vi "SM_AI-DAQInstrument.vi"(7 "AI TaskName":string, 8 "error in (no error)":errorcluster, 11 "DAQ Process AppData":T1) -> (0 "error out":errorcluster)   [LabVIEW 2022 SP3, in "DAQ.lvclass"]
doc: "Developed by Kevin Thompson\nkevin@thompsonengineering.net\n\nCopyright 2018-2020\nThompson Engineering, LLC"
uses:
  DAQ.lvclass
  Process_DAQ SM AppData--cluster.ctl
  DataTypes/TD DAQ Settings--cluster.ctl
  DataTypes/TD DI Instrument Settings--cluster.ctl
  DataTypes/TD AI Instrument Settings--cluster.ctl
  DataTypes/TD AI InstSettings--cluster.ctl
  TD SimAI Ranges--cluster.ctl
  <vilib>/TELLC/Dynamic CVT API/TD Dynamic CVT DVR--ref.ctl
  Support/DataQueues/DataTypes/DataQ SelectType--enum.ctl
  DAQ.lvclass/DAQ.ctl
  TD local raw AI Data--cluster.ctl
  DataTypes/AsyncMsg_DAQ--enum.ctl
  DataTypes/TD DaqState--enum.ctl
  <vilib>/DAQmx/read.llb/DAQmx Read (Analog 2D DBL NChan NSamp).vi
  Accessors/Get Dependency.vi
  Util/CONST AI TaskIO KeyName.vi
  <vilib>/TELLC/Dynamic CVT API/Get Dynamic CVT Data.vi
  <vilib>/DAQmx/miscellaneous.llb/DAQmx Fill In Error Info.vi
  Support/DataQueues/DataQueues.lvclass
  DAQ_Common/Lib/ErrorHandler/ErrorHandler.lvclass
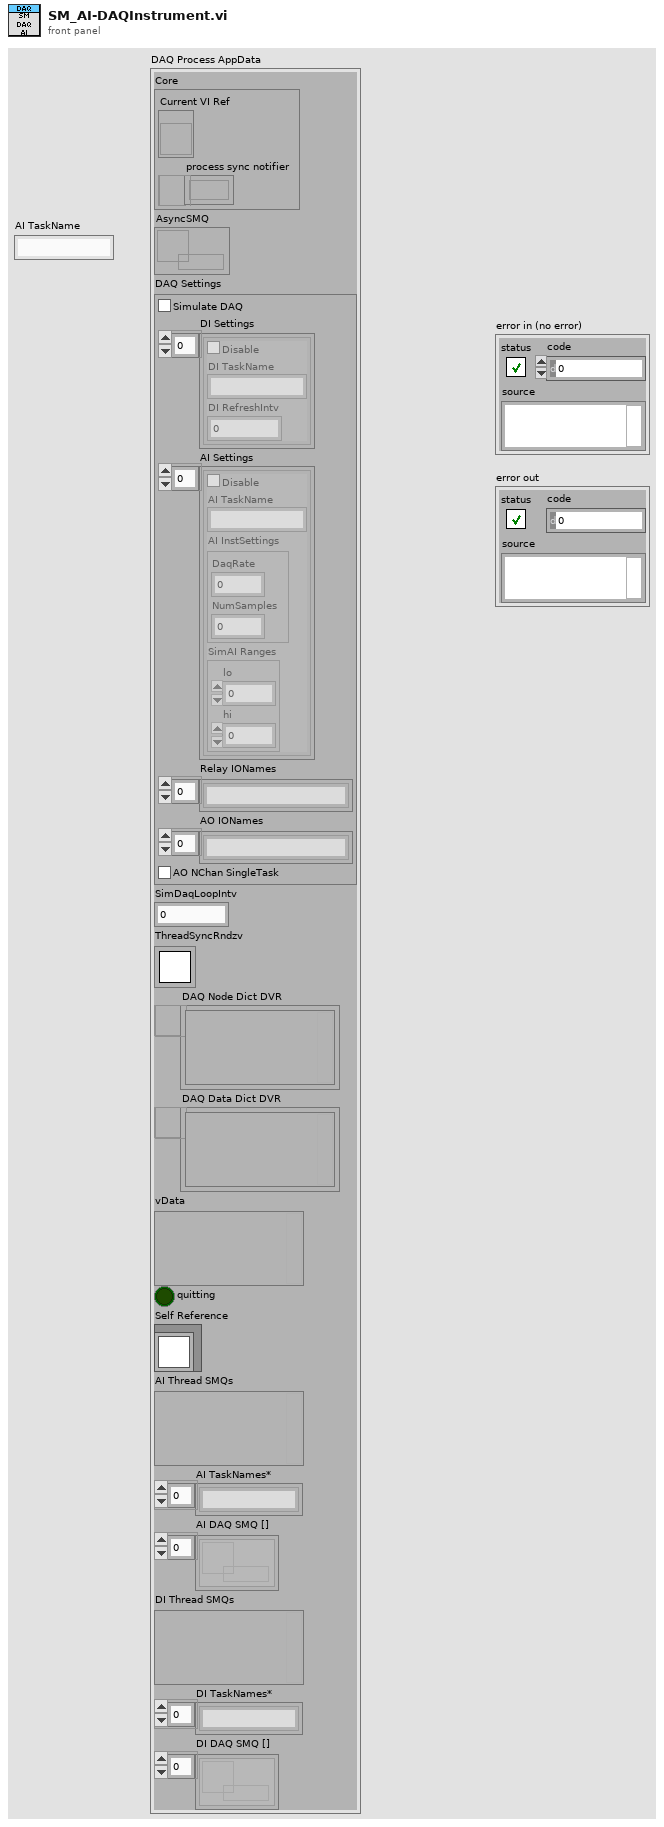
[diagram p1: front panel]
types:
  T1 = typedef "DAQ.lvclass/Process_DAQ SM AppData--cluster.ctl" = cluster{"Core":cluster{"Current VI Ref":refnum<vi>, "process sync notifier":refnum<notifier>}, "AsyncSMQ":refnum<queue>, "DAQ Settings":T2, "SimDaqLoopIntv":i32, "ThreadSyncRndzv":T7, "DAQ Node Dict DVR":T8, "DAQ Data Dict DVR":T8, "vData":variant, "quitting":bool, "Self Reference":refnum<class "DAQ.lvclass">, "AI Thread SMQs":variant, "AI TaskNames*":string[], "AI DAQ SMQ []":refnum<queue>[], "DI Thread SMQs":variant, "DI TaskNames*":string[], "DI DAQ SMQ []":refnum<queue>[]}
  T2 = typedef "DAQ.lvclass/TD DAQ Settings--cluster.ctl" = cluster{"Simulate DAQ":bool, "DI Settings":T3[], "AI Settings":T4[], "Relay IONames":string[], "AO IONames":string[], "AO NChan SingleTask":bool}
  T3 = typedef "DAQ.lvclass/TD DI Instrument Settings--cluster.ctl" = cluster{"Disable":bool, "DI TaskName":string, "DI RefreshIntv":i32}
  T4 = typedef "DAQ.lvclass/TD AI Instrument Settings--cluster.ctl" = cluster{"Disable":bool, "AI TaskName":string, "AI InstSettings":T5, "SimAI Ranges":T6}
  T5 = typedef "DAQ.lvclass/TD AI InstSettings--cluster.ctl" = cluster{"DaqRate":dbl, "NumSamples":i32}
  T6 = typedef "DAQ.lvclass/TD SimAI Ranges--cluster.ctl" = cluster{"lo":dbl, "hi":dbl}
  T7 = typedef "Rendezvous RefNum" = refnum<k1>
  T8 = typedef "TD Dynamic CVT DVR--ref.ctl" = refnum<data-value>
  T9 = enum32{"Invalid", "Standard", "Closed", "Hidden", "Minimized", "Maximized"}
  T10 = cluster{"UpdateUIControl Ev":refnum<user-event>, "stop process Ev":refnum<user-event>, "change mode Ev":refnum<user-event>}
  T11 = typedef "DataQueues.lvclass/DataQ SelectType--enum.ctl" = enum16{"MainProcess", "LogEngine", "LocalDAQThread"}
  T12 = typedef "DAQ.lvclass/TD local raw AI Data--cluster.ctl" = cluster{"TimeStamp_(s)":dbl, "data":dbl[][]}
  T13 = typedef "DAQ.lvclass/AsyncMsg_DAQ--enum.ctl" = enum16{"DAQ.SendAI_InstSettings"}
  T14 = typedef "DAQ.lvclass/TD DaqState--enum.ctl" = enum16{"Unknown", "Stopped", "Running", "Error"}
  T15 = typedef "DAQ.lvclass/TD AI local thread params--clustser.ctl" = cluster{"AI IONames":string[], "DAQ running":bool, "RawAIDataQ":T16, "AI Local CmdQ":refnum<queue>, "AI TaskName":string, "AI SMQ":refnum<queue>, "AI Settings":T4, "MainProc_ScanDataQ":T17, "Logger_ScanDataQ":T17, "DAQ Task Start Time":timestamp}
  T16 = typedef "DataQueues.lvclass/Analog DataSet MultiRow--QRef.ctl" = refnum<queue>
  T17 = typedef "DataQueues.lvclass/Analog DataSet MultiRow & ChanNames--QRef.ctl" = refnum<queue>
  T18 = cluster{"DAQ Process AppData":T1, "AI thread params":T15}
  T19 = typedef "Type Descriptor Enumeration__ogtk.ctl" = enum8{"<Null>", "I8", "I16", "I32", "I64", "U8", "U16", "U32", "U64", "SGL", "DBL", "EXT", "CSG", "CDB", "CXT", "0x0F", "0x10", "0x11", "0x12", "0x13", "0x14", "Enum U8", "Enum U16", "Enum U32", "Enum U64", "SGL PQ", "DBL PQ", "EXT PQ", "CSG PQ", "CDB PQ", "CXT PQ", "0x1F", "0x20", "Boolean", "0x22", "0x23", "0x24", "0x25", "0x26", "0x27", "0x28", "0x29", "0x2A", "0x2B", "0x2C", "0x2D", "0x2E", "0x2F", "String", "0x31", "Path", "Pict", "0x34", "0x35", "0x36", "DAQ", "0x38", "0x39", "0x3A", "0x3B", "0x3C", "0x3D", "0x3E", "0x3F", "Array", "0x41", "0x42", "0x43", "0x44", "0x45", "0x46", "0x47", "0x48", "0x49", "0x4A", "0x4B", "0x4C", "0x4D", "0x4E", "0x4F", "Cluster", "0x51", "0x52", "Variant", "Waveform", "0x55", "0x56", "0x57", "0x58", "0x59", "0x5A", "0x5B", "0x5C", "0x5D", "0x5E", "Fixed Point", "0x60", "0x61", "0x62", "0x63", "0x64", "0x65", "0x66", "0x67", "0x68", "0x69", "0x6A", "0x6B", "0x6C", "0x6D", "0x6E", "0x6F", "Refnum", "0x71", "0x72", "Set Collection", "Map Collection"}
  T20 = typedef "DAQ.lvclass/TD DAQ Device--enum.ctl" = enum16{"DI", "DO", "AIVolt", "AICurr", "AILoRes", "AO"}
  T21 = typedef "DAQ.lvclass/Dependency--cluster.ctl" = cluster{"DataQueues":refnum<class "DataQueues.lvclass">}
  T22 = cluster{"AI InstSettings":T5, "AI TaskName":string}
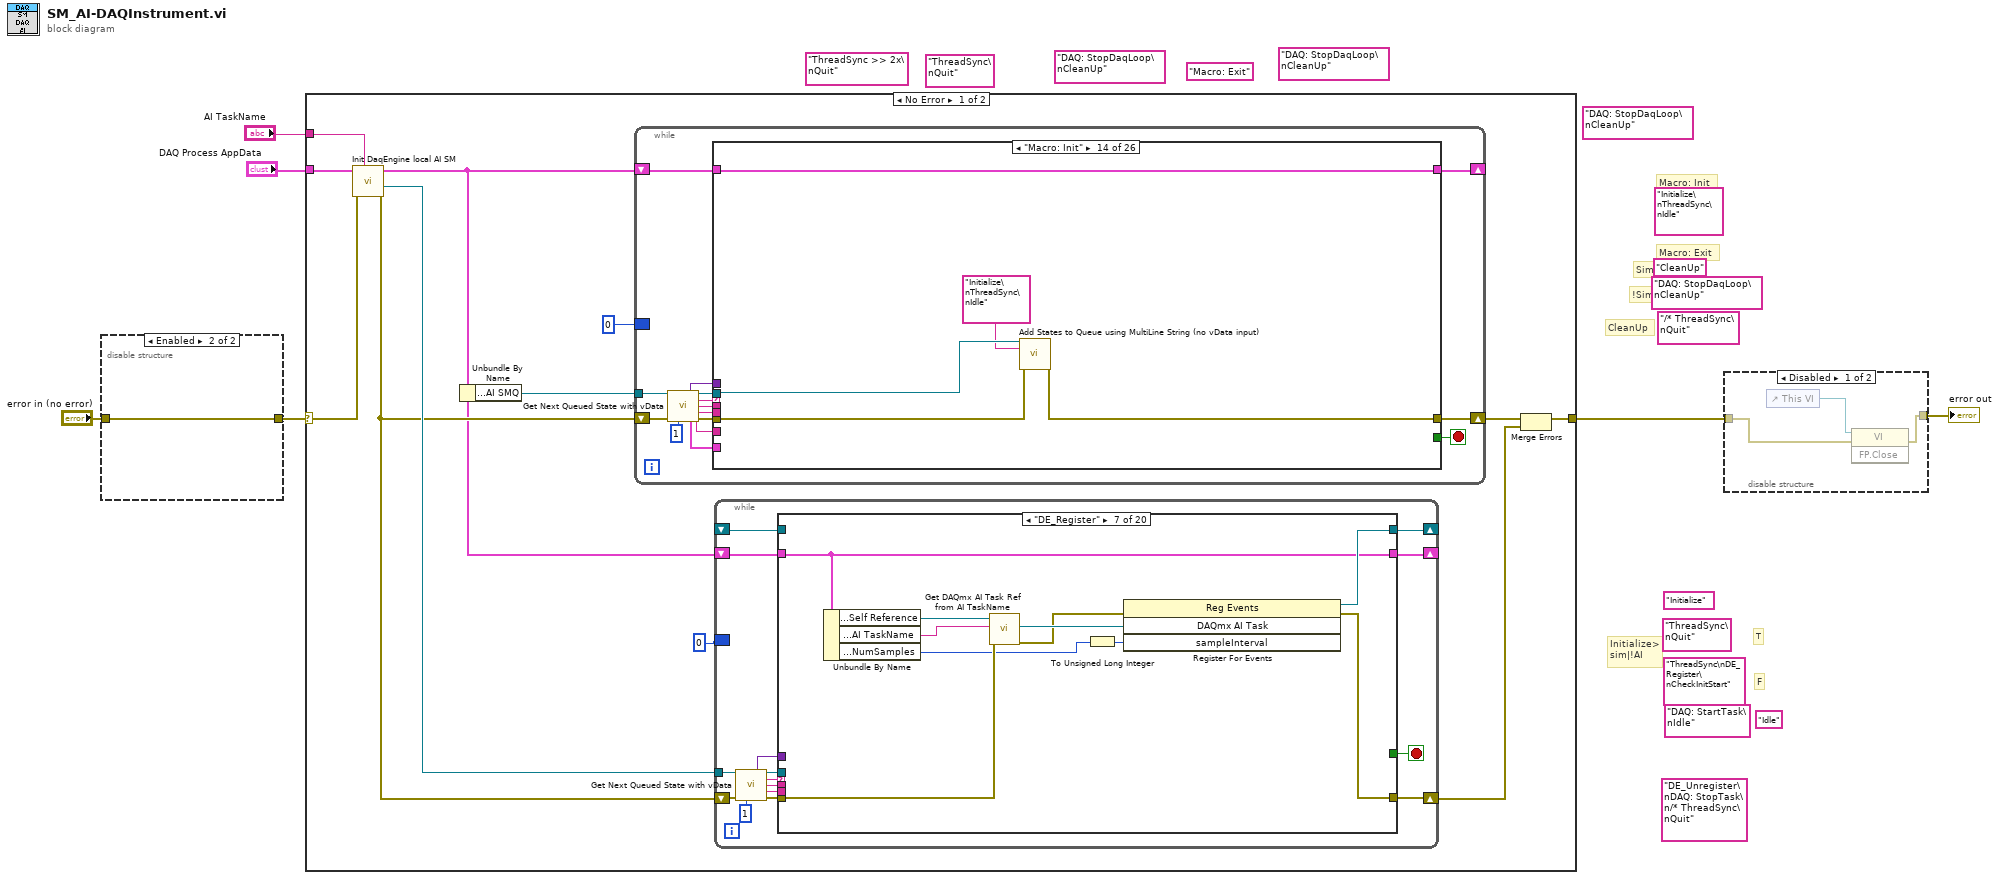
[diagram p0: block diagram]
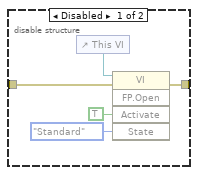
[diagram p3: hidden frame]
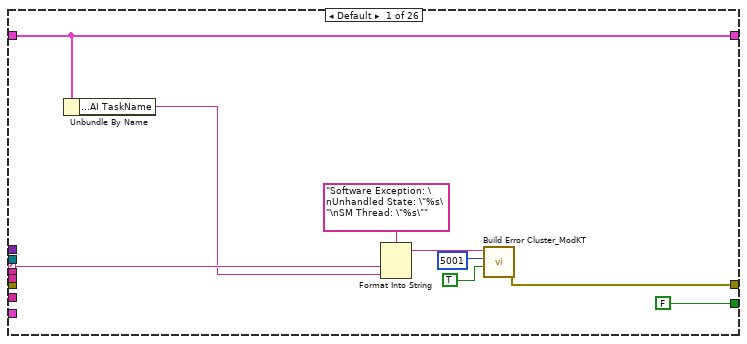
[diagram p4: hidden frame]
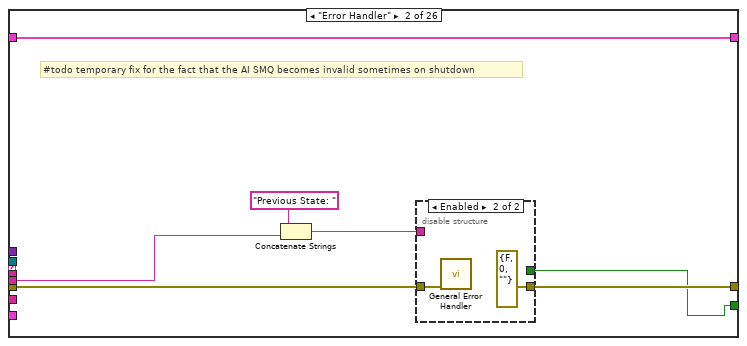
[diagram p5: hidden frame]
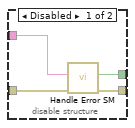
[diagram p6: hidden frame]
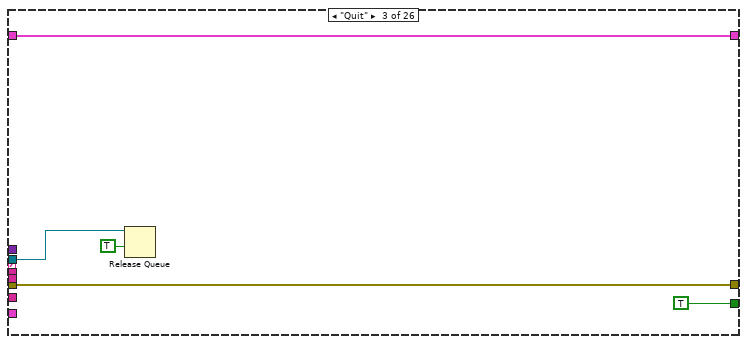
[diagram p7: hidden frame]
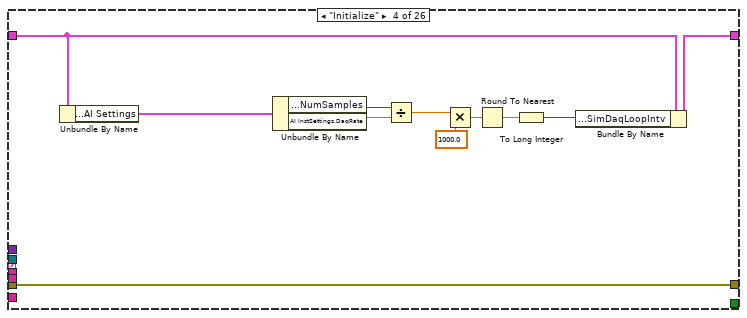
[diagram p8: hidden frame]
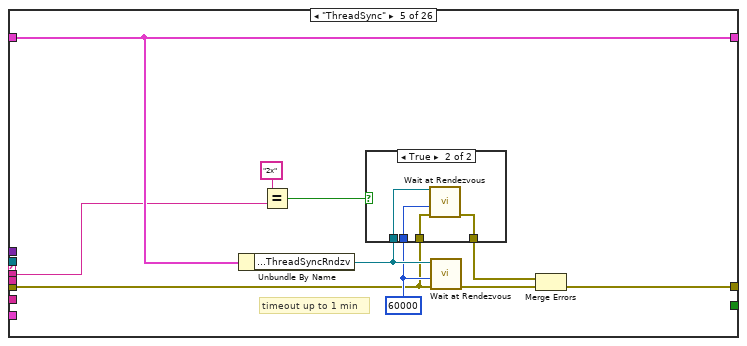
[diagram p9: hidden frame]
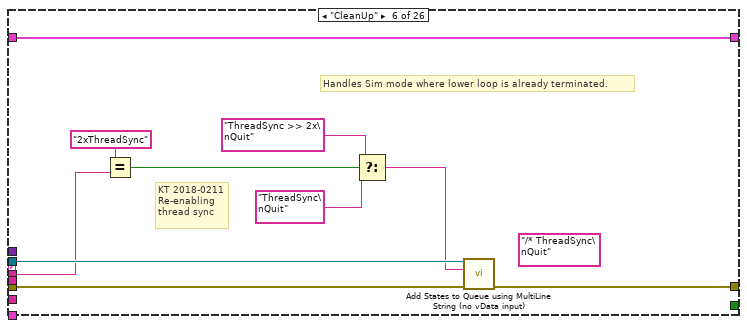
[diagram p11: hidden frame]
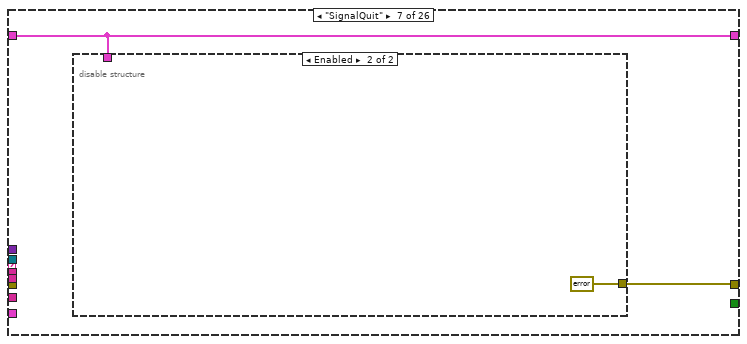
[diagram p12: hidden frame]
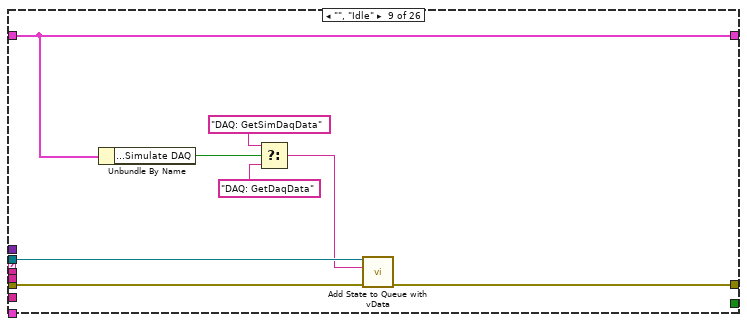
[diagram p15: hidden frame]
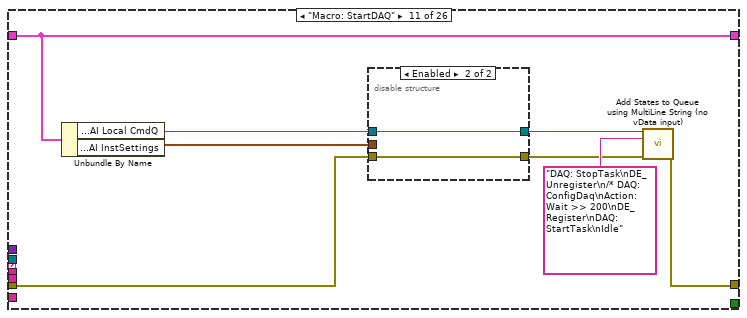
[diagram p17: hidden frame]
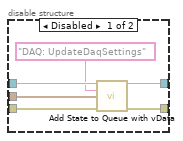
[diagram p18: hidden frame]
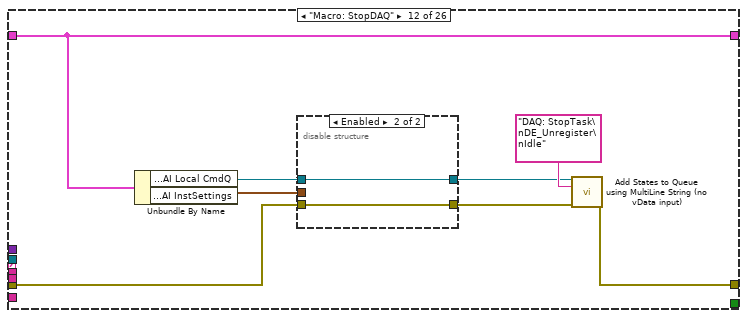
[diagram p19: hidden frame]
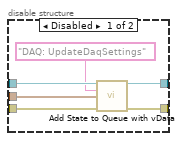
[diagram p20: hidden frame]
diagram:
  (unwired) "ThreadSync >> 2x\nQuit" ("states in")
  (unwired) "ThreadSync\nQuit" ("states in")
  (unwired) "DAQ: StopDaqLoop\nCleanUp"
  (unwired) "Macro: Exit"
  (unwired) "DAQ: StopDaqLoop\nCleanUp"
  (unwired) "DAQ: StopDaqLoop\nCleanUp"
  (unwired) "Idle"
  (unwired) "DAQ: StartTask\nIdle"
  (unwired) "ThreadSync\nDE_Register\nCheckInitStart"
  (unwired) "DE_Unregister\nDAQ: StopTask\n/* ThreadSync\nQuit" ("states in")
  (unwired) "Initialize" ("states in")
  (unwired) "ThreadSync\nQuit"
  (unwired) "/* ThreadSync\nQuit" ("states in")
  (unwired) "DAQ: StopDaqLoop\nCleanUp"
  (unwired) "CleanUp"
  (unwired) "Initialize\nThreadSync\nIdle"
  # "F"
  # "T"
  # "Initialize>\nsim|!AI"
  # "CleanUp"
  # "!Sim"
  # "Sim"
  # "Macro: Init"
  # "Macro: Exit"
  n1 = disable-structure shown="Enabled" {
    disable-tunnel: "error in (no error)" -> [w8 w12]
    disable-tunnel: [w7 w12] -> w1
    frame Disabled {
      n2 = control-ref of="This VI"() -> (w11:refnum<vi>)
      n3 = invoke class="VI" method="FP.Open"(reference=w11, error in=w8, "Activate"=TRUE ("Activate?"), "State"=T9."Standard") -> (error out=w7:errorcluster)  [unwired: 1 in, 4 out]
    }
    frame Enabled {
    }
  }
  n4 = case shown="No Error" w1 {
    selector: w1 -> [w22 w615]
    tunnel: [w20 w615] -> w4
    tunnel: "DAQ Process AppData" -> [w16 _]
    tunnel: "AI TaskName" -> [w15 _]
    frame No Error {
      n5 = call "Init DaqEngine local AI SM.vi"("AI TaskName"=w15, "error in (no error)"=w22, "DAQ Process AppData"=w16) -> ("error out"=w21:errorcluster, "local LoopCmdQ"=w23:refnum<queue>, "DaqProces AI AppData+"=w17:T18)  [unwired: 6 in]
      n6 = Unbundle By Name(w17) -> ("AI thread params.AI SMQ"=w14:refnum<queue>)
      n7 = while {
        shift-right: [w29] -> _
        shift-left: w17 -> [w38]
        shift-right: [w32] -> w24
        shift-left: w21 -> [w31]
        tunnel: w14 -> [w28]
        border: u32 0 -> [_]
        stop <- w34 stop-if-true
        n8 = call <vilib>:"Get Next Queued State with vData.vi"("queue in"=w28, "error in (no error)"=w31, "timeout (100)"=1) -> ("vData out"=w35:variant, "queue out"=w30:refnum<queue>, "Next State"=w37:string, "queued msg"=w36:string, "Prev State"=w25:string, "RemainingElements"=w27:cluster{"state":string, "vData":variant}[], "error out"=w33:errorcluster)  [unwired: 6 in]
        n9 = case shown="\"Macro: Init\"" w37 {
          selector: w37 -> [w42 _ _ _ _ _ _ _ _ _ _ _ _ _ _ _ _ _ _ _ _ _ _ _ _ _]
          tunnel: w38 -> [w40 w54 w65 w75 w86 w101 w102 w106 w113 w117 w118 w134 w155 w186 w193 w202 w228 w231 w235 w248 w260 w316 w320 w327 w328 w333]
          tunnel: w36 -> [_ _ _ _ w78 w97 _ _ _ _ _ _ _ _ _ _ _ _ _ _ _ _ _ w326 _ _]
          tunnel: w35 -> [_ _ _ _ _ _ _ _ _ _ _ _ w151 _ _ w203 _ _ _ _ _ _ _ _ w331 w336]
          tunnel: w25 -> [_ _ _ _ _ _ _ _ _ _ _ _ _ _ _ _ _ _ _ _ _ _ _ _ _ _]
          tunnel: [FALSE w48 TRUE _ _ _ _ _ _ _ _ _ _ _ _ _ _ _ _ _ _ _ _ _ _ _] -> w34
          tunnel: w33 -> [_ w51 w64 w67 w82 w99 _ w107 w112 w116 w120 w135 w152 w189 w194 w199 w227 w232 w245 w247 w273 w317 w319 w321 w330 w337]
          tunnel: [w41 w49 w64 w67 w81 w100 w103 w107 w114 w116 w119 w136 w153 w187 w195 w200 w227 w233 w245 w246 w272 w315 w319 w322 w329 w335] -> w32
          tunnel: w30 -> [_ _ w61 _ _ w98 _ _ w115 _ _ _ _ w188 w196 w204 _ _ _ _ _ _ _ _ _ _]
          tunnel: [w40 w54 w65 w76 w86 w101 w102 w106 w113 w117 w118 w134 w154 w186 w193 w201 w228 w231 w244 w248 w260 w316 w320 w327 w328 w334] -> w29
          tunnel: w27 -> [_ _ _ _ _ _ _ _ _ _ _ _ _ _ _ _ _ _ _ _ _ _ _ _ _ _]
          tunnel: w25 -> [_ w50 _ _ _ _ _ _ _ _ _ _ _ _ _ _ _ _ _ _ _ _ _ _ _ _]
          frame Default {
            n10 = Unbundle By Name(w40) -> ("AI thread params.AI TaskName"=w39:string)
            n11 = Format Into String(format string="Software Exception: \nUnhandled State: \"%s\"\nSM Thread: \"%s\"", w42, w39) -> (resulting string=w43:string)  [unwired: 2 in, 1 out]
            n12 = call <vilib>:"Build Error Cluster_ModKT .vi"("Prepend String (\"\")"=w43, "code"=5001, "error? (F)"=TRUE ("error?")) -> ("error out"=w41:errorcluster)  [unwired: 4 in, 1 out]
          }
          frame "Error Handler" {
            # "#todo temporary fix for the fact that the AI SMQ becomes invalid sometimes on shutdown"
            n13 = Concatenate Strings("Previous State: ", w50) -> (w53:string)
            n14 = disable-structure shown="Enabled" {
              disable-tunnel: w53 -> [w58 _]
              disable-tunnel: w51 -> [w57 w60]
              disable-tunnel: [w56 errorcluster {"status"=FALSE, "code"=0, "source"=""} ("error constant")] -> w49
              disable-tunnel: [w55 _] -> w48
              frame Disabled {
                n15 = call "Handle Error SM.vi"("error in (no error)"=w57, "CustomMessage"=w58) -> ("error out"=w56:errorcluster, "Shutdown?"=w55:bool)  [unwired: 7 in, 1 out]
              }
              frame Enabled {
                n16 = call <vilib>:"General Error Handler.vi"("error in (no error)"=w60) -> ()  [unwired: 10 in, 5 out]
              }
            }
          }
          frame "Quit" {
            n17 = Release Queue(queue=w61, force destroy? (F)=TRUE) -> ()  [unwired: 1 in, 3 out]
          }
          frame "Initialize" {
            n18 = Unbundle By Name(w75) -> ("AI thread params.AI Settings"=w66:T4)
            n19 = Unbundle By Name(w66) -> ("AI InstSettings.NumSamples"=w69:i32, "AI InstSettings.DaqRate"=w68:dbl)
            n20 = Divide(x=w69, y=w68) -> (x/y=w71:dbl)
            n21 = Multiply(x=w71, y=1000.0) -> (x*y=w74:dbl)
            n22 = Round To Nearest(number=w74) -> (nearest integer value=w72:dbl)
            n23 = To Long Integer(number=w72) -> (32bit integer=w70:i32)
            n24 = Bundle By Name(cluster=w75, "DAQ Process AppData.SimDaqLoopIntv"=w70) -> (w76:T18)
          }
          frame "ThreadSync" {
            w83 = 60000 ("ms timeout (-1)")
            # "timeout up to 1 min"
            n25 = Unbundle By Name(w86) -> ("DAQ Process AppData.ThreadSyncRndzv"=w84:T7)
            n26 = Equal?(x="2x", y=w78) -> (x = y?=w77:bool)
            n27 = case shown="True" w77 {
              tunnel: w84 -> [_ w91]
              tunnel: w83 -> [_ w90]
              tunnel: w82 -> [w87 w89]
              tunnel: [w87 w88] -> w80
              frame False {
              }
              frame True {
                n28 = call <vilib>:"Wait at Rendezvous.vi"("error in (no error)"=w89, "ms timeout (-1)"=w90, "rendezvous"=w91) -> ("error out"=w88:errorcluster)  [unwired: 2 in, 2 out]
              }
            }
            n29 = call <vilib>:"Wait at Rendezvous.vi"("error in (no error)"=w82, "ms timeout (-1)"=w83, "rendezvous"=w84) -> ("error out"=w85:errorcluster)  [unwired: 2 in, 2 out]
            n30 = Merge Errors(w80, w85) -> (w81:errorcluster)
          }
          frame "CleanUp" {
            (unwired) "/* ThreadSync\nQuit" ("states in")
            # "Handles Sim mode where lower loop is already terminated."
            # "KT 2018-0211\nRe-enabling\nthread sync"
            n31 = Equal?(x="2xThreadSync", y=w97) -> (x = y?=w95:bool)
            n32 = Select(t="ThreadSync >> 2x\nQuit" ("states in"), s=w95, f="ThreadSync\nQuit" ("states in")) -> (s? t:f=w92:string)
            n33 = call <vilib>:"Add States to Queue using MultiLine String (no vData input).vi"("queue in"=w98, "states in"=w92, "error in"=w99) -> ("error out"=w100:errorcluster)  [unwired: 10 in, 2 out]
          }
          frame "SignalQuit" {
            n34 = disable-structure shown="Enabled" {
              disable-tunnel: [w104 errorcluster {"status"=FALSE, "code"=0, "source"=""} ("error constant")] -> w103
              disable-tunnel: w102 -> [_ _]
              frame Disabled {
              }
              frame Enabled {
              }
            }
          }
          frame "CheckTimer" {
            # "NoOp"
          }
          frame "", "Idle" {
            n35 = Unbundle By Name(w113) -> ("DAQ Process AppData.DAQ Settings.Simulate DAQ"=w111:bool)
            n36 = Select(t="DAQ: GetSimDaqData" ("state"), s=w111, f="DAQ: GetDaqData" ("state")) -> (s? t:f=w108:string)
            n37 = call <vilib>:"Add State to Queue with vData.vi"("queue in"=w115, "state in"=w108, "error in"=w112) -> ("error out"=w114:errorcluster)  [unwired: 9 in, 3 out]
          }
          frame "------ Macro ------" {
          }
          frame "Macro: StartDAQ" {
            n38 = Unbundle By Name(w118) -> ("AI thread params.AI Local CmdQ"=w124:refnum<queue>, "AI thread params.AI Settings.AI InstSettings"=w125:T5)
            n39 = disable-structure shown="Enabled" {
              disable-tunnel: w124 -> [w131 w133]
              disable-tunnel: w125 -> [w129 _]
              disable-tunnel: [w128 w133] -> w121
              disable-tunnel: [w127 w132] -> w122
              disable-tunnel: w120 -> [w126 w132]
              frame Disabled {
                n40 = call <vilib>:"Add State to Queue with vData.vi"("queue in"=w131, "state in"="DAQ: UpdateDaqSettings", "vData (\"\")"=w129, "error in"=w126) -> ("queue out"=w128:refnum<queue>, "error out"=w127:errorcluster)  [unwired: 8 in, 2 out]
              }
              frame Enabled {
              }
            }
            n41 = call <vilib>:"Add States to Queue using MultiLine String (no vData input).vi"("queue in"=w121, "states in"="DAQ: StopTask\nDE_Unregister\n/* DAQ: ConfigDaq\nAction: Wait >> 200\nDE_Register\nDAQ: StartTask\nIdle", "error in"=w122) -> ("error out"=w119:errorcluster)  [unwired: 10 in, 2 out]
          }
          frame "Macro: StopDAQ" {
            n42 = Unbundle By Name(w134) -> ("AI thread params.AI Local CmdQ"=w141:refnum<queue>, "AI thread params.AI Settings.AI InstSettings"=w137:T5)
            n43 = disable-structure shown="Enabled" {
              disable-tunnel: w141 -> [w147 w149]
              disable-tunnel: w137 -> [w145 _]
              disable-tunnel: [w144 w149] -> w138
              disable-tunnel: [w143 w148] -> w139
              disable-tunnel: w135 -> [w142 w148]
              frame Disabled {
                n44 = call <vilib>:"Add State to Queue with vData.vi"("queue in"=w147, "state in"="DAQ: UpdateDaqSettings", "vData (\"\")"=w145, "error in"=w142) -> ("queue out"=w144:refnum<queue>, "error out"=w143:errorcluster)  [unwired: 8 in, 2 out]
              }
              frame Enabled {
              }
            }
            n45 = call <vilib>:"Add States to Queue using MultiLine String (no vData input).vi"("queue in"=w138, "states in"="DAQ: StopTask\nDE_Unregister\nIdle", "error in"=w139) -> ("error out"=w136:errorcluster)  [unwired: 10 in, 2 out]
          }
          frame "Macro: CfgDAQ" {
            # "#NOTE: KT 2019-0713\nRe-Config of DAQ settings is presently disabled."
            # "#TODO: will need to update\nAI InstSettings values here and\ntransferred to other places since\nthose values are used in other\nareas of the application"
            # "From external command\n(e.g. sequencer)"
            # "From DAQ Configuration"
            # "#TODO:  finish implementing\nStartDaq params to reconfigure\nDAQ settings (sample rate / num samples)"
            n46 = Unbundle By Name(w155) -> ("AI thread params.AI Local CmdQ"=w159:refnum<queue>, "AI thread params.AI Settings.AI InstSettings"=w162:T5)
            n47 = call <userlib>:"Get TDEnum from Data__ogtk.vi"("Data"=w151) -> ("Type Descriptor Enumeration"=w161:T19)  [unwired: 4 in]
            n48 = case shown="\"Cluster\"" w161 {
              tunnel: w152 -> [w168 w176]
              tunnel: [w168 w175] -> w160
              tunnel: w151 -> [_ w174]
              tunnel: w162 -> [w167 w170]
              tunnel: [w167 w171] -> w150
              frame "<Null>", Default {
              }
              frame "Cluster" {
                w173 = T5 {"DaqRate"=-1.0, "NumSamples"=-1} ("AI InstSettings")
                n49 = Variant To Data(error in=w176, type=w173, Variant=w174) -> (data=w172:T5, error out=w175:errorcluster)
                n50 = Equal?(x=w173, y=w172) -> (x = y?=w169:bool)
                n51 = Select(t=w170, s=w169, f=w172) -> (s? t:f=w171:T5)
              }
            }
            n52 = disable-structure shown="Enabled" {
              disable-tunnel: w159 -> [w182 w184]
              disable-tunnel: w150 -> [w180 _]
              disable-tunnel: [w179 w184] -> w156
              disable-tunnel: [w178 w183] -> w157
              disable-tunnel: w160 -> [w177 w183]
              frame Enabled {
                n53 = call <vilib>:"Add State to Queue with vData.vi"("queue in"=w182, "state in"="DAQ: UpdateDaqSettings", "vData (\"\")"=w180, "error in"=w177) -> ("queue out"=w179:refnum<queue>, "error out"=w178:errorcluster)  [unwired: 8 in, 2 out]
              }
              frame Disabled {
              }
            }
            n54 = disable-structure shown="Enabled" {
              disable-tunnel: w155 -> [w165 w166]
              disable-tunnel: [w164 w166] -> w154
              disable-tunnel: w150 -> [w163 _]
              frame Enabled {
                n55 = Bundle By Name(cluster=w165, "AI thread params.AI Settings.AI InstSettings"=w163) -> (w164:T18)
              }
              frame Disabled {
              }
            }
            n56 = call <vilib>:"Add States to Queue using MultiLine String (no vData input).vi"("queue in"=w156, "states in"="DAQ: StopTask\nDE_Unregister\nDAQ: ConfigDaq\nAction: Wait >> 200\nDE_Register\nDAQ: StartTask\nIdle", "error in"=w157) -> ("error out"=w153:errorcluster)  [unwired: 10 in, 2 out]
          }
          frame "Macro: Init" {
            n57 = call <vilib>:"Add States to Queue using MultiLine String (no vData input).vi"("queue in"=w188, "states in"="Initialize\nThreadSync\nIdle", "error in"=w189) -> ("error out"=w187:errorcluster)  [unwired: 10 in, 2 out]
          }
          frame "Macro: Exit" {
            # "error here indicates lower loop\nis already terminated"
            n58 = Unbundle By Name(w193) -> ("AI thread params.AI Local CmdQ"=w192:refnum<queue>)
            n59 = Get Queue Status(queue=w192) -> (error out=w191:errorcluster)  [unwired: 2 in, 7 out]
            n60 = case shown="No Error" w191 {
              tunnel: ["DAQ: StopDaqLoop\nCleanUp" "CleanUp >> 2xThreadSync"] -> w190
              frame No Error {
              }
              frame Error {
              }
            }
            n61 = call <vilib>:"Add States to Queue using MultiLine String (no vData input).vi"("queue in"=w196, "states in"=w190, "error in"=w194) -> ("error out"=w195:errorcluster)  [unwired: 10 in, 2 out]
          }
          frame "Macro: UpdateDaqSettings" {
            n62 = disable-structure shown="Enabled" {
              disable-tunnel: w204 -> [w218 _]
              disable-tunnel: w203 -> [_ _]
              disable-tunnel: w202 -> [w217 w226]
              disable-tunnel: [w216 w226] -> w201
              disable-tunnel: [w208 w225] -> w200
              disable-tunnel: w199 -> [w206 w225]
              frame Disabled {
                n63 = Bundle By Name(cluster=w217) -> (w216:T18)  [unwired: 1 in]
                n64 = Get Queue Status() -> (error out=w219:errorcluster)  [unwired: 3 in, 7 out]
                n65 = Equal?() -> (x=w214:dbl, y=w215:dbl, x = y?=w211:bool)
                n66 = case shown="No Error" w219 {
                  tunnel: [w221 ""] -> w213
                  tunnel: w211 -> [w220 _]
                  frame No Error {
                    n67 = case shown="True" w220 {
                      tunnel: ["" "DAQ: SendDaqUpdate"] -> w221
                      frame False {
                      }
                      frame True {
                      }
                    }
                  }
                  frame Error {
                    # "data collection loop is\nterminated if in sim mode"
                  }
                }
                n68 = Empty String/Path?(string/path=w213) -> (empty?=w212:bool)
                n69 = call <vilib>:"Add State to Queue with vData.vi"("queue in"=w218, "state in"=w213, "bypass (F)"=w212) -> ("queue out"=w207:refnum<queue>, "error in"=w205:errorcluster, "error out"=w209:errorcluster)  [unwired: 8 in, 2 out]
                n70 = call <vilib>:"Add States to Queue using MultiLine String (no vData input).vi"("queue in"=w207, "states in"="DAQ: SetSimDaqLoopIntv", "error in"=w209) -> ("error out"=w208:errorcluster)  [unwired: 10 in, 2 out]
              }
              frame Enabled {
                # "#NOTE: presently no plans to allow DAQ reconfigure while operating.\nDAQ settings are read once from config at startup.  App restart required\nto change settings (sampling rate, num samples, etc.)."
              }
            }
          }
          frame "------ DAQ ------" {
          }
          frame "DAQ: StopDaqLoop" {
            n71 = Unbundle By Name(w231) -> ("AI thread params.AI Local CmdQ"=w230:refnum<queue>)
            n72 = call <vilib>:"Add States to Queue using MultiLine String (no vData input).vi"("queue in"=w230, "states in"="Macro: Exit", "error in"=w232) -> ("error out"=w233:errorcluster)  [unwired: 10 in, 2 out]
          }
          frame "DAQ: SetSimDaqLoopIntv" {
            # "This case would only be called if we allow DAQ settings updates\nduring operation.  Currently no plans to allow that."
            n73 = Unbundle By Name(w235) -> ("DAQ Process AppData.DAQ Settings.AI Settings"=w236:T4[])
            n74 = Index Array(array=w236) -> (element=w234:T4)  [unwired: 1 in]
            n75 = Unbundle By Name(w234) -> ("AI InstSettings.NumSamples"=w238:i32, "AI InstSettings.DaqRate"=w237:dbl)
            n76 = Divide(x=w238, y=w237) -> (x/y=w240:dbl)
            n77 = Multiply(x=w240, y=1000.0) -> (x*y=w243:dbl)
            n78 = Round To Nearest(number=w243) -> (nearest integer value=w241:dbl)
            n79 = To Long Integer(number=w241) -> (32bit integer=w239:i32)
            n80 = Bundle By Name(cluster=w235, "DAQ Process AppData.SimDaqLoopIntv"=w239) -> (w244:T18)
          }
          frame "DAQ: SendDaqUpdate" {
            n81 = disable-structure shown="Disabled" {
              disable-tunnel: w248 -> [w257 _]
              disable-tunnel: w247 -> [w251 w258]
              disable-tunnel: [w250 w258] -> w246
              frame Disabled {
                n82 = Unbundle By Name(w257) -> ("AI thread params.AI Local CmdQ"=w256:refnum<queue>, "AI thread params.AI Settings.AI InstSettings"=w254:T5)
                n83 = call <vilib>:"Add State to Queue with vData.vi"("queue in"=w256, "state in"="DAQ: UpdateDaqSettings", "vData (\"\")"=w254, "error in"=w251) -> ("queue out"=w253:refnum<queue>, "error out"=w252:errorcluster)  [unwired: 8 in, 2 out]
                n84 = call <vilib>:"Add States to Queue using MultiLine String (no vData input).vi"("queue in"=w253, "states in"="DAQ: StopTask\nDE_Unregister\nDAQ: ConfigDaq\nDE_Register\nDAQ: StartTask\nIdle", "error in"=w252) -> ("error out"=w250:errorcluster)  [unwired: 10 in, 2 out]
              }
              frame Enabled {
                # "#NOTE: presently no plans to allow DAQ reconfigure while operating.\nDAQ settings are read once from config at startup.  App restart required\nto change settings (sampling rate, num samples, etc.)."
              }
            }
          }
          frame "DAQ: GetDaqData" {
            # "#todo check this"
            # "#TODO: remove and replace"
            n85 = Unbundle By Name(w260) -> ("AI thread params.RawAIDataQ"=w271:T16)  [unwired: 1 out]
            n86 = Unbundle By Name(w260) -> ("AI thread params.MainProc_ScanDataQ"=w261:T17, "AI thread params.AI TaskName"=w263:string, "DAQ Process AppData.DAQ Node Dict DVR"=w265:T8, "DAQ Process AppData.DAQ Data Dict DVR"=w266:T8, "AI thread params.AI IONames"=w267:string[])
            n87 = Unbundle By Name(w260) -> ("AI thread params.Logger_ScanDataQ"=w259:T17)
            n88 = Get Queue Status(queue=w271, error in (no error)=w273) -> (queue out=w270:T16, error out=w268:errorcluster, # elements in queue=w264:i32)  [unwired: 1 in, 5 out]
            n89 = Greater Than 0?(x=w264) -> (x > 0?=w269:bool)
            n90 = case shown="False" w269 {
              tunnel: w270 -> [_ w287]
              tunnel: w268 -> [w276 w286]
              tunnel: w267 -> [_ w283]
              tunnel: w266 -> [_ w284]
              tunnel: w265 -> [_ w285]
              tunnel: [w275 w282] -> w272
              tunnel: w264 -> [_ w281]
              tunnel: w263 -> [_ w280]
              tunnel: T10 {"UpdateUIControl Ev"=refnum, "stop process Ev"=refnum, "change mode Ev"=refnum} ("Public P&ID Events") -> [_ w279]
              tunnel: w261 -> [_ w278]
              tunnel: w259 -> [_ w277]
              frame False {
                n91 = call <userlib>:"Wait (ms)__ogtk.vi"("error in (no error)"=w276, "milliseconds to wait"=u32 50 ("wait (ms)")) -> ("error out"=w275:errorcluster)  [unwired: 8 in, 1 out]
              }
              frame True {
                n92 = for {
                  N: w281 -> [_]
                  tunnel: w287 -> [w297]
                  shift-right: [w295] -> w282
                  shift-left: w286 -> [w296]
                  tunnel: w285 -> [w294]
                  tunnel: w284 -> [w293]
                  tunnel: w283 -> [w292]
                  tunnel: w280 -> [w291]
                  tunnel: w279 -> [w290]
                  tunnel: w278 -> [w289]
                  tunnel: w277 -> [w288]
                  n93 = call "Read AI DAQ Data.vi"("DAQ Node Dict DVR"=w294, "AI TaskName"=w291, "Public P&ID Events"=w290, "MainProc_ScanDataQ"=w289, "DAQ Data Dict DVR"=w293, "AI IONames"=w292, "RawAIDataQ"=w297, "error in"=w296, "Logger_ScanDataQ"=w288) -> ("error out"=w295:errorcluster)  [unwired: 4 in, 2 out]
                }
              }
            }
          }
          frame "DAQ: GetSimDaqData" {
            # "compensate for state machine\nidle timeout (1 ms)"
            n94 = Unbundle By Name(w316) -> ("AI thread params.AI TaskName"=w300:string, "AI thread params.Logger_ScanDataQ"=w299:T17, "AI thread params.MainProc_ScanDataQ"=w298:T17, "DAQ Process AppData.DAQ Node Dict DVR"=w313:T8, "DAQ Process AppData.DAQ Data Dict DVR"=w312:T8, "AI thread params.AI IONames"=w303:string[], "AI thread params.AI Settings.SimAI Ranges"=w301:T6, "DAQ Process AppData.SimDaqLoopIntv"=w302:i32)
            n95 = Subtract(x=w302, y=u32 1) -> (x-y=w308:u32)
            n96 = In Range and Coerce(upper limit=u32 10000, x=w308, lower limit=u32 1) -> (coerced(x)=w307:u32)  [unwired: 1 out]
            n97 = call <userlib>:"Wait (ms)__ogtk.vi"("error in (no error)"=w317, "milliseconds to wait"=w307) -> ("error out"=w314:errorcluster)  [unwired: 8 in, 1 out]
            n98 = call "Sim Read AI DAQ Data.vi"("DAQ Node Dict DVR"=w313, "IP_RawDataQ"=w298, "TDMS_RawDataQ"=w299, "AI TaskName"=w300, "DAQ Data Dict DVR"=w312, "AI IONames"=w303, "SimAI Ranges"=w301, "error in"=w314) -> ("error out"=w315:errorcluster)  [unwired: 5 in, 2 out]
            n99 = stacked-sequence {
              tunnel: [w318] -> w304
              tunnel: w315 -> [_]
              frame #0 {
                n100 = Tick Count (ms)() -> (millisecond timer value=w318:u32)
              }
            }
            n101 = feedback #1() -> (w311:u32)
            n102 = feedback-in #1(w304) -> ()
            n103 = Subtract(x=w304, y=w311) -> (x-y=w310:u32)
            n104 = call "Update DaqLoopTimer Q.vi"("elapsed time (ms)"=w310, "AI TaskName"=w300) -> ()  [unwired: 6 in]
          }
          frame "------ Action ------" {
          }
          frame "Action: Wait" {
            n105 = Scan From String(format string="%d", input string=w326) -> (output 1=w324:i32)  [unwired: 3 in, 3 out]
            n106 = To Unsigned Long Integer(number=w324) -> (unsigned 32bit integer=w323:u32)
            n107 = call <userlib>:"Wait (ms)__ogtk.vi"("error in (no error)"=w321, "milliseconds to wait"=w323) -> ("error out"=w322:errorcluster)  [unwired: 8 in, 1 out]
          }
          frame "Action: UpdateInterval" {
            # "Not applicable to AI DAQ"
            n108 = Variant To Data(error in=w330, type=0.0, Variant=w331) -> (error out=w329:errorcluster)  [unwired: 1 out]
          }
          frame "Action: UpdateEnable" {
            n109 = disable-structure shown="Disabled" {
              disable-tunnel: w337 -> [w350 w353]
              disable-tunnel: w336 -> [w348 _]
              disable-tunnel: [w345 w353] -> w335
              disable-tunnel: [w341 w354] -> w334
              disable-tunnel: w333 -> [w340 w354]
              frame Disabled {
                n110 = Unbundle By Name(w340) -> ("DaqDev"=w339:T20)
                n111 = Variant To Data(error in=w350, type=TRUE, Variant=w348) -> (data=w338:bool, error out=w346:errorcluster)
                n112 = case shown="\"DI\"" w339 {
                  tunnel: w340 -> [w352 _ _]
                  tunnel: [w352 _ _] -> w341
                  tunnel: w338 -> [_ _ _]
                  frame Default {
                  }
                  frame "DI" {
                  }
                  frame "DI" {
                  }
                }
                n113 = Unbundle By Name(w341) -> ("AI thread params.AI Local CmdQ"=w349:refnum<queue>, "DAQ Process AppData.DAQ Settings.Simulate DAQ"=w342:bool)
                n114 = Select(t="DAQ: StartTask", s=w338, f="DAQ: StopTask") -> (s? t:f=w343:string)
                n115 = call <vilib>:"Add State to Queue with vData.vi"("queue in"=w349, "state in"=w343, "bypass (F)"=w342, "error in"=w346) -> ("error out"=w345:errorcluster)  [unwired: 8 in, 3 out]
              }
              frame Enabled {
              }
            }
          }
        }
      }
      n116 = while {
        shift-right: [w365] -> _
        shift-left: _ -> [w364]
        shift-right: [w363] -> _
        shift-left: w17 -> [w369]
        shift-right: [w362] -> w19
        shift-left: w21 -> [w367]
        tunnel: w23 -> [w368]
        border: u32 0 -> [_]
        stop <- w356 stop-if-true
        n117 = call <vilib>:"Get Next Queued State with vData.vi"("queue in"=w368, "error in (no error)"=w367, "timeout (100)"=1) -> ("vData out"=w355:variant, "queue out"=w360:refnum<queue>, "Next State"=w359:string, "queued msg"=w358:string, "Prev State"=w357:string, "error out"=w366:errorcluster)  [unwired: 6 in, 1 out]
        n118 = case shown="\"DE_Register\"" w359 {
          selector: w359 -> [w373 _ _ _ _ _ _ _ _ _ _ _ _ _ _ _ _ _ _ _]
          tunnel: w369 -> [w371 w385 w396 w407 w419 w433 w445 w451 w456 w492 w498 w503 w506 w511 w525 w549 w576 w593 w601 w603]
          tunnel: w366 -> [_ w381 w404 w415 w424 w432 w441 w449 w457 w491 w496 _ w505 w509 w524 w550 w575 w592 w597 w606]
          tunnel: [w378 w386 w405 w416 w425 w436 w446 w450 w454 w493 w499 w504 w507 w513 w526 w555 w580 w594 w602 w608] -> w365
          tunnel: w364 -> [w378 w386 w405 w416 w425 w436 _ w450 w454 w493 w499 w504 w507 w513 w526 w555 w580 w594 w602 w608]
          tunnel: [w371 w385 w396 w406 w419 w433 w445 w451 w455 w492 w498 w503 w506 w510 w525 w552 w577 w593 w601 w604] -> w363
          tunnel: [w372 w382 w404 w414 w423 w431 w444 w447 w452 w491 w495 w501 w505 w508 w523 w551 w574 w592 w595 w605] -> w362
          tunnel: w360 -> [_ _ _ w413 w422 _ _ _ _ _ w494 w502 _ _ _ _ _ _ _ _]
          tunnel: w358 -> [_ _ _ _ _ _ _ _ _ _ _ _ _ _ _ _ _ _ w596 _]
          tunnel: w357 -> [_ w380 _ _ _ _ _ _ _ _ _ _ _ _ _ _ _ _ _ _]
          tunnel: [_ w379 TRUE _ _ _ _ _ _ _ _ _ _ _ _ _ _ _ _ _] -> w356
          tunnel: w355 -> [_ _ _ _ _ _ _ _ _ _ _ _ _ w512 _ _ _ _ _ w607]
          frame Default {
            n119 = Unbundle By Name(w371) -> ("AI thread params.AI TaskName"=w370:string)
            n120 = Format Into String(format string="Software Exception: \nUnhandled State: \"%s\"\nSM Thread: \"%s\"", w373, w370) -> (resulting string=w377:string)  [unwired: 2 in, 1 out]
            n121 = call <vilib>:"Build Error Cluster_ModKT .vi"("Prepend String (\"\")"=w377, "code"=5001, "error? (F)"=TRUE ("error?")) -> ("error out"=w372:errorcluster)  [unwired: 4 in, 1 out]
          }
          frame "Error Handler" {
            (unwired) "DE_Unregister\nDAQ: StopTask\nThreadSync\nQuit" ("states in")
            # "#todo temporary fix for the fact that the AI SMQ becomes invalid sometimes on shutdown"
            n122 = Concatenate Strings("Previous State: ", w380) -> (w383:string)
            n123 = disable-structure shown="Enabled" {
              disable-tunnel: w383 -> [w390 _]
              disable-tunnel: [w389 errorcluster {"status"=FALSE, "code"=0, "source"=""} ("error constant")] -> w382
              disable-tunnel: w381 -> [w388 w392]
              disable-tunnel: [w387 _] -> w379
              frame Disabled {
                n124 = call "Handle Error SM.vi"("error in (no error)"=w388, "CustomMessage"=w390) -> ("error out"=w389:errorcluster, "Shutdown?"=w387:bool)  [unwired: 7 in, 1 out]
              }
              frame Enabled {
                n125 = call <vilib>:"General Error Handler.vi"("error in (no error)"=w392) -> ()  [unwired: 10 in, 5 out]
              }
            }
          }
          frame "Exit", "Quit" {
            n126 = Unbundle By Name(w396) -> ("AI thread params.AI Local CmdQ"=w402:refnum<queue>, "DAQ Process AppData.Self Reference"=w400:refnum<class "DAQ.lvclass">)
            n127 = Unbundle By Name(w396) -> ("AI thread params.AI TaskName"=w395:string)
            n128 = property class="DAQ"(reference=w400) -> ("Accessors:Dependency"=w394:T21)  [unwired: 1 in, 2 out]
            n129 = Release Queue(queue=w402, force destroy? (F)=TRUE) -> (error out=w397:errorcluster)  [unwired: 1 in, 2 out]
            n130 = Unbundle By Name(w394) -> ("DataQueues"=w393:refnum<class "DataQueues.lvclass">)
            n131 = call <userlib>:"Clear All Errors__ogtk.vi"("Error In"=w397) -> ()  [unwired: 3 in, 1 out]
            n132 = call "Destroy DataQ.vi"("Select"=DataQ_SelectType--enum."LocalDAQThread", "TaskName"=w395, "DataQueues in"=w393) -> ("error out"=w398:errorcluster)  [unwired: 6 in, 2 out]
            n133 = call <userlib>:"Clear All Errors__ogtk.vi"("Error In"=w398) -> ()  [unwired: 3 in, 1 out]
          }
          frame "Initialize" {
            # "quit this loop if simulate mode, or not an AI thread"
            n134 = Unbundle By Name(w407) -> ("DAQ Process AppData.DAQ Settings.Simulate DAQ"=w409:bool)
            n135 = Select(t="ThreadSync\nQuit", s=w409, f="ThreadSync\nDE_Register\nCheckInitStart") -> (s? t:f=w411:string)
            n136 = call <vilib>:"Add States to Queue using MultiLine String (no vData input).vi"("queue in"=w413, "states in"=w411, "error in"=w415) -> ("error out"=w414:errorcluster)  [unwired: 10 in, 2 out]
            n137 = Bundle By Name(cluster=w407, "AI thread params.DAQ running"=FALSE) -> (w406:T18)
          }
          frame "CheckInitStart" {
            n138 = disable-structure shown="Enabled" {
              disable-tunnel: w419 -> [w428 _]
              disable-tunnel: [w426 TRUE ("TCAI")] -> w418
              frame Disabled {
                n139 = Unbundle By Name(w428) -> ("DaqDev"=w427:T20)
                n140 = case shown="Default" w427 {
                  tunnel: [FALSE _ _] -> w426
                  frame Default {
                  }
                  frame "DI" {
                  }
                  frame "DI" {
                  }
                }
              }
              frame Enabled {
              }
            }
            n141 = Select(t="/* DAQ: StartTask\nIdle", s=w418, f="Idle") -> (s? t:f=w421:string)
            n142 = call <vilib>:"Add States to Queue using MultiLine String (no vData input).vi"("queue in"=w422, "states in"=w421, "error in"=w424) -> ("error out"=w423:errorcluster)  [unwired: 10 in, 2 out]
          }
          frame "ThreadSync" {
            # "timeout up to 1 min"
            n143 = Unbundle By Name(w433) -> ("DAQ Process AppData.ThreadSyncRndzv"=w434:T7)
            n144 = call <vilib>:"Wait at Rendezvous.vi"("error in (no error)"=w432, "ms timeout (-1)"=60000, "rendezvous"=w434) -> ("error out"=w431:errorcluster)  [unwired: 2 in, 2 out]
          }
          frame "DE_Register" {
            n145 = Unbundle By Name(w445) -> ("DAQ Process AppData.Self Reference"=w442:refnum<class "DAQ.lvclass">, "AI thread params.AI TaskName"=w440:string, "AI thread params.AI Settings.AI InstSettings.NumSamples"=w437:i32)
            n146 = call "Get DAQmx AI Task Ref from AI TaskName.vi"("error in (no error)"=w441, "AI TaskName"=w440, "DAQ"=w442) -> ("error out"=w438:errorcluster, "DAQmx AI Task"=w439:refnum<k21>)  [unwired: 6 in, 1 out]
            n147 = To Unsigned Long Integer(number=w437) -> (unsigned 32bit integer=w443:u32)
            n148 = register-events(error in=w438, w439, w443) -> (reference out=w446:refnum<event-registration>, error out=w444:errorcluster)  [unwired: 1 in]
          }
          frame "DE_Unregister" {
            n149 = Unregister For Events(event registration refnum=w450, error in=w449) -> (error out=w448:errorcluster)
            n150 = call <userlib>:"Clear All Errors__ogtk.vi"("Error In"=w448) -> ("Error Out"=w447:errorcluster)  [unwired: 3 in]
          }
          frame "", "EventHandler", "Idle" {
            n151 = event shown="[0] Timeout" {
              selector: w454 -> [_ _]
              dyn-events: _ -> [_ _]
              timeout: 5 -> [_ _]
              tunnel: w457 -> [w460 w483]
              tunnel: w456 -> [w461 w472]
              tunnel: [w461 w472] -> w455
              tunnel: [w459 w478] -> w452
              event Timeout {
                n152 = event-data() -> ()  [unwired: 1 in, 3 out]
                n153 = Unbundle By Name(w461) -> ("AI thread params.DAQ running"=w458:bool)
                n154 = case shown="True" w458 {
                  tunnel: w460 -> [w464 w465]
                  tunnel: [w463 w465] -> w459
                  frame False {
                    n155 = call <userlib>:"Wait (ms)__ogtk.vi"("error in (no error)"=w464, "milliseconds to wait"=u32 1000 ("wait (ms)")) -> ("error out"=w463:errorcluster)  [unwired: 8 in, 1 out]
                  }
                  frame True {
                  }
                }
              }
              event Every N Samples Acquired into Buffer {
                n156 = event-data() -> ("Time"=w476:i32, "CtlRef"=w484:refnum<k21>, "sampleInterval"=w486:u32)  [unwired: 1 in]
                n157 = Unbundle By Name(w472) -> ("AI thread params.RawAIDataQ"=w480:T16, "AI thread params.AI TaskName"=w471:string, "AI thread params.AI Settings.AI InstSettings.DaqRate"=w469:dbl, "AI thread params.AI Settings.AI InstSettings.NumSamples"=w470:i32)
                n158 = stacked-sequence {
                  tunnel: w486 -> [w489]
                  tunnel: [w487] -> w485
                  tunnel: [w488] -> w468
                  frame #0 {
                    n159 = Get Date/Time In Seconds() -> (seconds since 1Jan1904=w490:timestamp)
                    n160 = To Long Integer(number=w489) -> (32bit integer=w487:i32)
                    n161 = To Double Precision Float(number=w490) -> (double precision float=w488:dbl)
                  }
                }
                n162 = Divide(x=w470, y=w469) -> (x/y=w467:dbl)
                n163 = Subtract(x=w468, y=w467) -> (x-y=w466:dbl)
                n164 = To Unsigned Long Integer(number=w476) -> (unsigned 32bit integer=w473:u32)
                n165 = call-poly <vilib>:"DAQmx Read.vi"("task/channels in"=w484, "number of samples per channel"=w485, "error in"=w483) -> ("data"=w482:dbl[][], "error out"=w479:errorcluster)  [unwired: 10 in, 1 out]
                n166 = Bundle(cluster=T12 {"TimeStamp_(s)"=0.0, "data"=[]} ("output cluster"), "TimeStamp_(s)"=w466, "data"=w482) -> (w481:T12)
                n167 = feedback-in #2(w473) -> ()
                n168 = feedback #2() -> (w474:u32)
                n169 = Subtract(x=w473, y=w474) -> (x-y=w475:u32)
                n170 = call "Update DaqLoopTimer Q.vi"("elapsed time (ms)"=w475, "AI TaskName"=w471) -> ()  [unwired: 6 in]
                n171 = Enqueue Element(queue=w480, element=w481, error in (no error)=w479) -> (error out=w478:errorcluster)  [unwired: 1 in, 2 out]
              }
            }
          }
          frame "------ Macro ------" {
          }
          frame "Macro: Init" {
            n172 = call <vilib>:"Add States to Queue using MultiLine String (no vData input).vi"("queue in"=w494, "states in"="Initialize", "error in"=w496) -> ("error out"=w495:errorcluster)  [unwired: 10 in, 2 out]
          }
          frame "CleanUp", "Macro: Exit" {
            (unwired) "DE_Unregister\nDAQ: StopTask\n/* ThreadSync\nQuit" ("states in")
            # "KT 2018-0211\nRe-enabling\nthread sync"
            n173 = call <vilib>:"Add States to Queue using MultiLine String (no vData input).vi"("queue in"=w502, "states in"="DE_Unregister\nDAQ: StopTask\nThreadSync\nQuit") -> ("error out"=w501:errorcluster)  [unwired: 11 in, 2 out]
          }
          frame "------ DAQ ------" {
          }
          frame "DAQ: UpdateDaqSettings" {
            n174 = disable-structure shown="Enabled" {
              disable-tunnel: w512 -> [w520 _]
              disable-tunnel: w511 -> [w519 w522]
              disable-tunnel: [w518 w522] -> w510
              disable-tunnel: w509 -> [w516 w521]
              disable-tunnel: [w515 w521] -> w508
              frame Enabled {
                w514 = T5 {"DaqRate"=0.0, "NumSamples"=0}  # AI InstSettings
                n175 = Variant To Data(error in=w516, type=w514, Variant=w520) -> (data=w517:T5, error out=w515:errorcluster)
                n176 = Bundle By Name(cluster=w519, "AI thread params.AI Settings.AI InstSettings"=w517) -> (w518:T18)
              }
              frame Disabled {
              }
            }
          }
          frame "DAQ: ConfigDaq" {
            n177 = disable-structure shown="Enabled" {
              disable-tunnel: w525 -> [w543 _]
              disable-tunnel: w524 -> [w542 w547]
              disable-tunnel: [w539 w547] -> w523
              frame Enabled {
                w546 = 10123 items=["Finite Samples"=10178, "Continuous Samples"=10123] ("sample mode")
                n178 = Unbundle By Name(w543) -> ("DAQ Process AppData.Self Reference"=w531:refnum<class "DAQ.lvclass">, "AI thread params.AI TaskName"=w529:string, "AI thread params.AI Settings.AI InstSettings"=w535:T5)
                n179 = call <userlib>:"Wait (ms)__ogtk.vi"("error in (no error)"=w542, "milliseconds to wait"=u32 1500 ("wait (ms)")) -> ("error out"=w532:errorcluster)  [unwired: 8 in, 1 out]
                n180 = call "Get DAQmx AI Task Ref from AI TaskName.vi"("error in (no error)"=w532, "AI TaskName"=w529, "DAQ"=w531) -> ("error out"=w528:errorcluster, "DAQmx AI Task"=w527:refnum<k21>, "DAQ"=w530:refnum<class "DAQ.lvclass">)  [unwired: 6 in]
                n181 = Unbundle By Name(w535) -> ("DaqRate"=w538:dbl, "NumSamples"=w544:i32)
                n182 = Bundle("AI InstSettings"=w535, "AI TaskName"=w529) -> (w534:T22)  [unwired: 1 in]
                n183 = call "Config Chans Clock and Start Scanning.vi"("Rate"=w538, "stop&start now?"=FALSE ("start now?"), "sample mode"=w546, "error_in"=w528, "SamplesPerChan"=w544, "Task in"=w527) -> ("error_out"=w536:errorcluster)  [unwired: 4 in, 1 out]
                n184 = call "Generate AsyncMsg Event_DAQ.vi"("error in (no error)"=w536, "vData"=w534, "AsyncMsg"=AsyncMsg_DAQ--enum."DAQ.SendAI_InstSettings", "DAQ"=w530) -> ("error out"=w537:errorcluster)  [unwired: 6 in, 1 out]
                n185 = call <userlib>:"Wait (ms)__ogtk.vi"("error in (no error)"=w537, "milliseconds to wait"=u32 1500 ("wait (ms)")) -> ("error out"=w539:errorcluster)  [unwired: 8 in, 1 out]
              }
              frame Disabled {
              }
            }
          }
          frame "DAQ: StartTask" {
            n186 = Unbundle By Name(w549) -> ("AI thread params.DAQ running"=w554:bool)
            n187 = case shown="False" w554 {
              selector: w554 -> [_ w573]
              tunnel: [w569 w573] -> w553
              tunnel: w549 -> [w566 _]
              tunnel: w550 -> [w564 w572]
              tunnel: [w559 w572] -> w551
              tunnel: w549 -> [w557 w571]
              tunnel: [w556 w571] -> w548
              frame False {
                # "#todo this timestamp stored in right place? All thread pars instead?"
                n188 = Unbundle By Name(w566) -> ("DAQ Process AppData.Self Reference"=w568:refnum<class "DAQ.lvclass">, "AI thread params.AI TaskName"=w567:string)
                n189 = Get Date/Time In Seconds() -> (seconds since 1Jan1904=w558:timestamp)
                n190 = call "Get DAQmx AI Task Ref from AI TaskName.vi"("error in (no error)"=w564, "AI TaskName"=w567, "DAQ"=w568) -> ("error out"=w563:errorcluster, "DAQmx AI Task"=w565:refnum<k21>, "DAQ"=w562:refnum<class "DAQ.lvclass">)  [unwired: 6 in]
                n191 = call <vilib>:"DAQmx Start Task.vi"("task/channels in"=w565, "error in"=w563) -> ("error out"=w561:errorcluster)  [unwired: 12 in, 1 out]
                n192 = Bundle By Name(cluster=w557, "AI thread params.DAQ Task Start Time"=w558) -> (w556:T18)
                n193 = call "Fire DAQStateChanged Event_DAQ.vi"("error in (no error)"=w561, "DAQState"=TD_DaqState--enum."Running", "DAQ"=w562) -> ("error out"=w559:errorcluster)  [unwired: 7 in, 1 out]
                n194 = Unbundle By Name(w559) -> ("status"=w570:bool)
                n195 = Not(x=w570) -> (.not. x?=w569:bool)
              }
              frame True {
              }
            }
            n196 = Bundle By Name(cluster=w548, "AI thread params.DAQ running"=w553) -> (w552:T18)
          }
          frame "DAQ: StopTask" {
            n197 = Unbundle By Name(w576) -> ("AI thread params.DAQ running"=w579:bool)
            n198 = case shown="True" w579 {
              tunnel: [w581 w583] -> w574
              tunnel: w576 -> [_ w591]
              tunnel: w575 -> [w581 w587]
              frame False {
              }
              frame True {
                n199 = Unbundle By Name(w591) -> ("DAQ Process AppData.Self Reference"=w590:refnum<class "DAQ.lvclass">, "AI thread params.AI TaskName"=w588:string)
                n200 = call "Get DAQmx AI Task Ref from AI TaskName.vi"("error in (no error)"=w587, "AI TaskName"=w588, "DAQ"=w590) -> ("error out"=w586:errorcluster, "DAQmx AI Task"=w589:refnum<k21>, "DAQ"=w585:refnum<class "DAQ.lvclass">)  [unwired: 6 in]
                n201 = call <vilib>:"DAQmx Stop Task.vi"("task/channels in"=w589, "error in"=w586) -> ("error out"=w584:errorcluster)  [unwired: 12 in, 1 out]
                n202 = call "Fire DAQStateChanged Event_DAQ.vi"("error in (no error)"=w584, "DAQState"=TD_DaqState--enum."Stopped", "DAQ"=w585) -> ("error out"=w583:errorcluster)  [unwired: 7 in, 1 out]
              }
            }
            n203 = Bundle By Name(cluster=w576, "AI thread params.DAQ running"=FALSE) -> (w577:T18)
          }
          frame "------ Action ------" {
          }
          frame "Action: Wait" {
            n204 = Scan From String(format string="%d", input string=w596) -> (output 1=w599:i32)  [unwired: 3 in, 3 out]
            n205 = To Unsigned Long Integer(number=w599) -> (unsigned 32bit integer=w600:u32)
            n206 = call <userlib>:"Wait (ms)__ogtk.vi"("error in (no error)"=w597, "milliseconds to wait"=w600) -> ("error out"=w595:errorcluster)  [unwired: 8 in, 1 out]
          }
          frame "Action: SetInhibitErrDialog" {
            n207 = disable-structure shown="Enabled" {
              disable-tunnel: w607 -> [w611 _]
              disable-tunnel: w606 -> [w610 w614]
              disable-tunnel: [w609 w614] -> w605
              disable-tunnel: [_ w613] -> w604
              disable-tunnel: w603 -> [_ w613]
              frame Disabled {
                n208 = Variant To Data(error in=w610, type=TRUE, Variant=w611) -> (error out=w609:errorcluster)  [unwired: 1 out]
              }
              frame Enabled {
              }
            }
          }
        }
      }
      n209 = Merge Errors(w24, w19) -> (w20:errorcluster)
    }
    frame Error {
    }
  }
  n210 = disable-structure shown="Disabled" {
    disable-tunnel: w4 -> [w618 w619]
    disable-tunnel: [w616 w619] -> w3
    frame Disabled {
      n211 = control-ref of="This VI"() -> (w617:refnum<vi>)
      n212 = invoke class="VI" method="FP.Close"(reference=w617, error in=w618) -> (error out=w616:errorcluster)  [unwired: 1 in, 2 out]
    }
    frame Enabled {
    }
  }
  "error out" <- w3
